vi "Get stack cell d_voltage status_old.vi"(11 "Status Map":map{string, dbl}(c390)) -> (0 "Average":dbl format="%#_6f", 1 "Min":dbl, 2 "Max":dbl, 3 "Stack V":dbl)   [LabVIEW 2025]
uses:
  <userlib>/_MGI/1D Array/MGI Average/MGI Average (DBL[]).vi
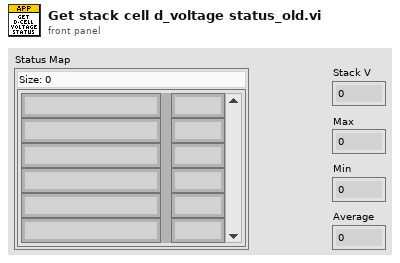
[diagram p1: front panel]
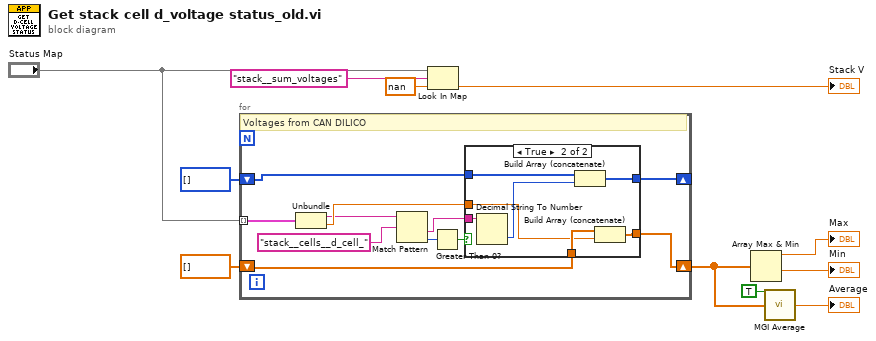
[diagram p0: block diagram]
diagram:
  n1 = for {
    tunnel: "Status Map" -> [w22] mode=indexing
    shift-right: [w13] -> _
    shift-left: i32[] [] -> [w12]
    shift-right: [w15] -> w1
    shift-left: dbl[] [] -> [w16]
    # "Voltages from CAN DILICO"
    n2 = Unbundle(w22) -> (w19:string, w20:dbl)
    n3 = Match Pattern(string=w19, regular expression="stack__cells__d_cell_") -> (after substring=w17:string, offset past match=w14:i32)  [unwired: 1 in, 2 out]
    n4 = Greater Than 0?(x=w14) -> (x > 0?=w21:bool)
    n5 = case shown="True" w21 {
      tunnel: w20 -> [_ w25]
      tunnel: w17 -> [_ w31]
      tunnel: w16 -> [w24 w30]
      tunnel: [w24 w29] -> w15
      tunnel: [w23 w27] -> w13
      tunnel: w12 -> [w23 w26]
      frame False {
      }
      frame True {
        n6 = Decimal String To Number(string=w31) -> (number=w28:i32)  [unwired: 2 in, 1 out]
        n7 = Build Array (concatenate)(w26, w28) -> (w27:i32[])
        n8 = Build Array (concatenate)(w30, w25) -> (w29:dbl[])
      }
    }
  }
  n9 = Look In Map(map="Status Map", key="stack__sum_voltages", default value=nan) -> (value=→"Stack V":dbl)  [unwired: 1 out]
  n10 = Array Max & Min(array=w1) -> (max value=→"Max":dbl, min value=→"Min":dbl)  [unwired: 2 out]
  n11 = call-poly <userlib>:"MGI Average.vi"("Double[]"=w1, "Ignore NaN? (F)"=TRUE) -> ("Average"=→"Average":dbl)
